vi "History Chart 1-Channel.vi"() -> ()   [LabVIEW 2016]
doc: "This VI re-creates the behavior of a History Chart with one channel.\nA template of this VI could be created to dynamically load as many history charts as needed.\n\nTo change the number of points in the graph, right-click the graph and select \"Chart History\nLength...\", then set the desired number of points."
uses:
  Nanonis Prog Interface.lvlib
panel:
  in  "Clear Chart":bool
  in  "stop":bool
  in  "Oversampling":i32=1 min=1 max=10000 step=1
  in  "Signal":i8(ring)
  out "Chart":sgl(graph)
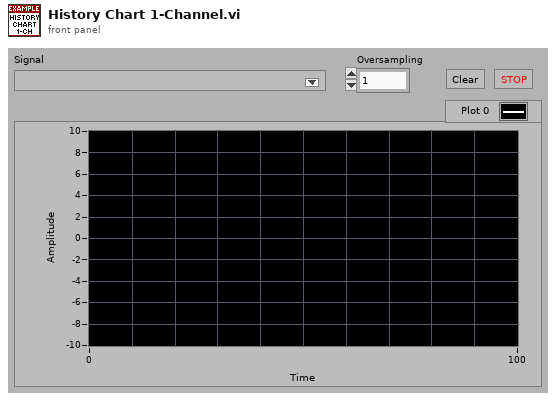
[diagram p1: front panel]
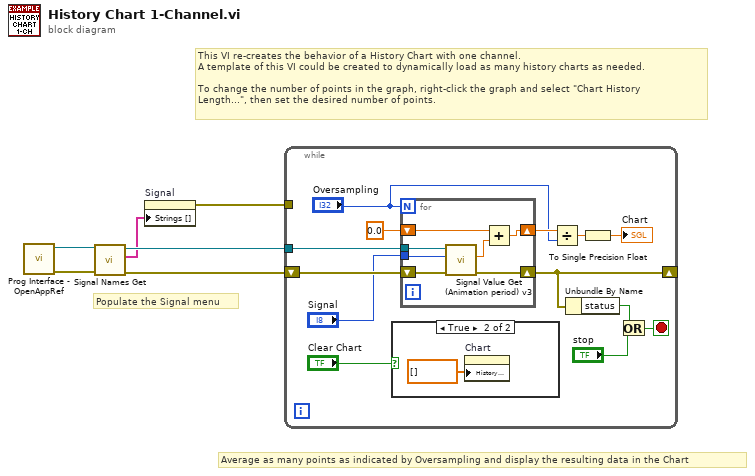
[diagram p0: block diagram]
diagram:
  # "This VI re-creates the behavior of a History Chart with one channel.\nA template of this VI could be created to dynamically load as many history charts as needed.\n\nTo change the number of points in the graph, right-click the graph and select \"Chart History\nLength...\", then set the desired number of points."
  # "Average as many points as indicated by Oversampling and display the resulting data in the Chart"
  # "Populate the Signal menu"
  n1 = call <userlib>:"Prog Interface - OpenAppRef.vi"() -> ("Error out"=w5:errorcluster, "Application reference"=w6:refnum<vi>)  [unwired: 6 in]
  n2 = call <userlib>:"Signal Names Get.vi"("error in (no error)"=w5, "Application ref in"=w6) -> ("error out"=w4:errorcluster, "Signals Names"=w2:string[], "Application ref out"=w3:refnum<vi>)  [unwired: 5 in]
  n3 = property on="Signal" class="Ring (strict)"("Strings []"=w2) -> (error out=w1:errorcluster)  [unwired: 2 in, 1 out]
  n4 = while {
    shift-right: [w11] -> _
    shift-left: w4 -> [w18]
    tunnel: w3 -> [w17]
    tunnel: w1 -> [_]
    stop <- w19 stop-if-true
    n5 = case shown="True" "Clear Chart" {
      frame False {
      }
      frame True {
        n6 = property on="Chart" class="WFChart (strict)"("History Data"=sgl[] []) -> ()  [unwired: 2 in, 2 out]
      }
    }
    n7 = for {
      N: "Oversampling" -> [_]
      shift-right: [w26] -> w11
      shift-left: w18 -> [w27]
      tunnel: w17 -> [w24]
      tunnel: "Signal" -> [w23]
      shift-right: [w21] -> w14
      shift-left: 0.0 ("x") -> [w22]
      n8 = call <userlib>:"Signal Value Get (Animation period) v3.vi"("error in (no error)"=w27, "Signal index (0-127)"=w23, "Application ref in"=w24) -> ("error out"=w26:errorcluster, "Signal value"=w25:sgl)  [unwired: 5 in, 1 out]
      n9 = Add(x=w22, y=w25) -> (x+y=w21:dbl)
    }
    n10 = Divide(x=w14, y="Oversampling") -> (x/y=w8:dbl)
    n11 = Unbundle By Name(w11) -> ("status"=w10:bool)
    n12 = To Single Precision Float(number=w8) -> (single precision float=→"Chart":sgl)
    n13 = Or(x=w10, y="stop") -> (x .or. y?=w19:bool)
  }
